vi "response.Has Error.vi"(8 "error in (no error)":errorcluster, 11 "Response in":refnum<class "Response.lvclass">) -> (0 "error out":errorcluster, 2 "error status":bool, 3 "Response out":refnum<class "Response.lvclass">)   [LabVIEW 2020, in "JSON-RPC Lib.lvlib" / "Response.lvclass"]
uses:
  Response.lvclass
  Response.lvclass/Response.ctl
  error/error.Read code.vi
  error/error.lvclass
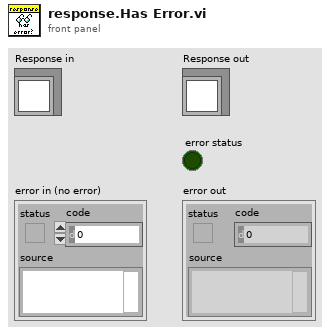
[diagram p1: front panel]
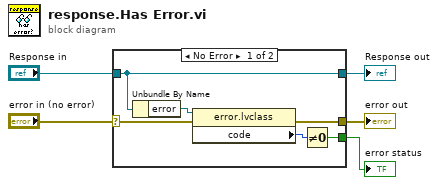
[diagram p0: block diagram]
diagram:
  n1 = case shown="No Error" "error in (no error)" {
    selector: "error in (no error)" -> [w7 w13]
    tunnel: [w6 w13] -> w4
    tunnel: [w11 w12] -> w2
    tunnel: "Response in" -> [w11 w12]
    tunnel: [w8 _] -> w1
    frame No Error {
      n2 = Unbundle By Name(w11) -> ("error"=w10:refnum<class "error.lvclass">)
      n3 = property class="error.lvclass"(reference=w10, error in=w7) -> (error out=w6:errorcluster, "code"=w9:i32)  [unwired: 1 out]
      n4 = Not Equal To 0?(x=w9) -> (x != 0?=w8:bool)
    }
    frame Error {
    }
  }
  "error out" <- w4
  "Response out" <- w2
  "error status" <- w1
